vi "Main Module.vi"(8 "Error In":errorcluster) -> (0 "Error Out":errorcluster)   [LabVIEW 2015, in "Entry Console.lvlib"]
uses:
  Entry Console.lvlib
  Public Controls/Wash steps selection buttons.ctl
  Private Controls/Module Data Cluster.ctl
  Private Controls/Module Action.ctl
  Controller/Controller.lvlib
panel:
  in  "Start":bool
  in  "Wash steps selection buttons":T1={"Under Body Wash"=FALSE, "Bug Remover"=FALSE, "Pre-Soak"=FALSE, "High Pressure Wash"=TRUE, "Low Pressure Wax"=FALSE, "Spot Free Rinse"=FALSE, "Tire Shine Foam"=FALSE, "Air Dry"=FALSE}
  # "[Covers: UI1]"
  # "[Covers: UI2]"
  # "[Covers: UI2A]"
  # "[Covers: UI2A1]"
  # "[Covers: UI2B]"
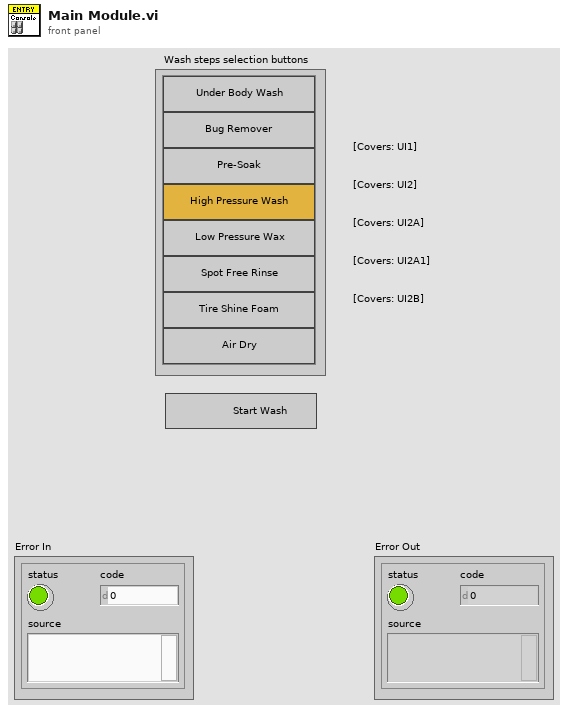
[diagram p1: front panel]
types:
  T1 = typedef "Entry Console.lvlib/Wash steps selection buttons.ctl" = cluster{"Under Body Wash":bool, "Bug Remover":bool, "Pre-Soak":bool, "High Pressure Wash":bool, "Low Pressure Wax":bool, "Spot Free Rinse":bool, "Tire Shine Foam":bool, "Air Dry":bool}
  T2 = typedef "Entry Console.lvlib/Module Data Cluster.ctl" = cluster{"Data":variant, "Action":T3}
  T3 = typedef "Entry Console.lvlib/Module Action.ctl" = enum16{"Init", "Close", "Error", "Start Wash"}
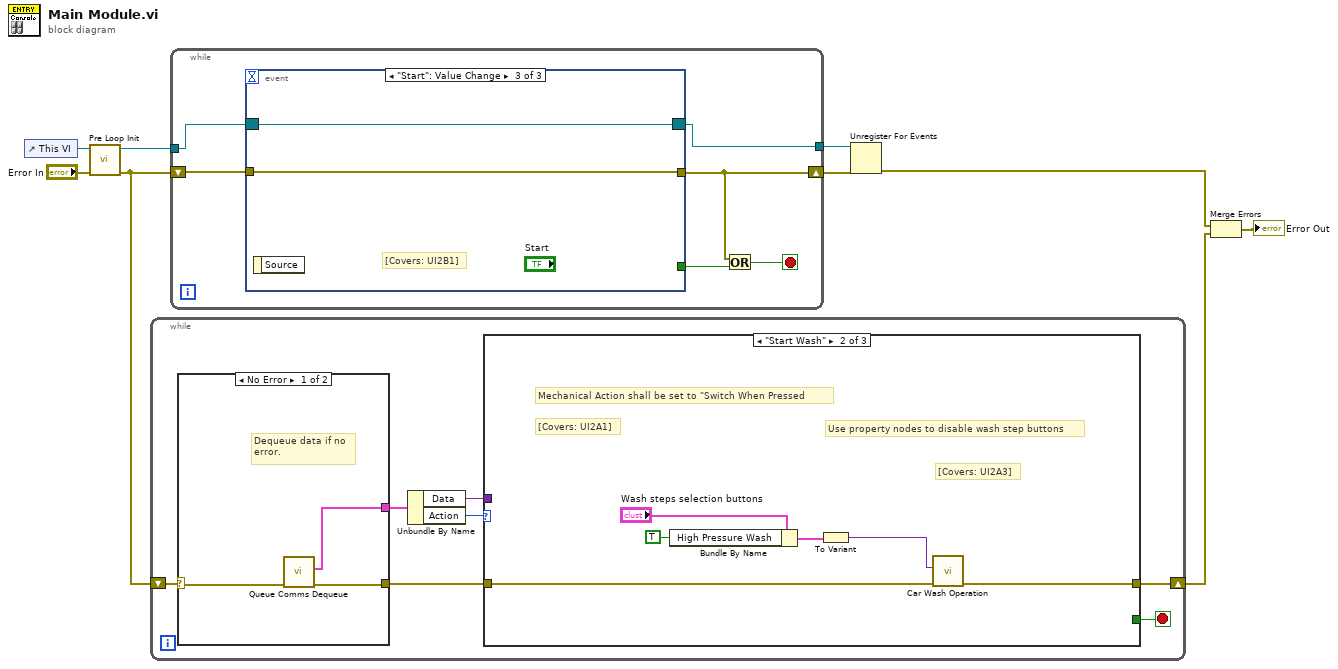
[diagram p0: block diagram]
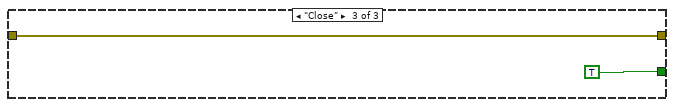
[diagram p3: hidden frame]
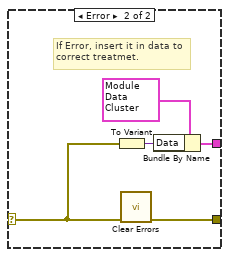
[diagram p4: hidden frame]
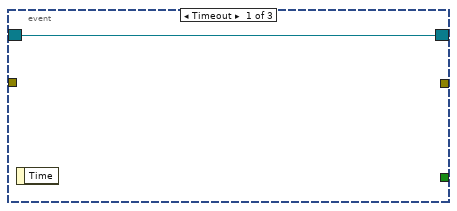
[diagram p5: hidden frame]
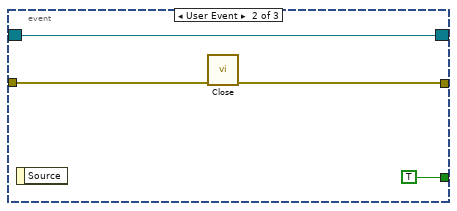
[diagram p6: hidden frame]
diagram:
  n1 = control-ref of="This VI"() -> (w8:refnum<vi>)
  n2 = call "Pre Loop Init.vi"("Error In"="Error In", "This VI"=w8) -> ("Error Out"=w4:errorcluster, "Event Registration Refnum"=w7:refnum<event-registration>)  [unwired: 8 in]
  n3 = while {
    shift-right: [w10] -> w2
    shift-left: w4 -> [w16]
    stop <- w11 stop-if-true
    n4 = case shown="No Error" w16 {
      selector: w16 -> [w28 w31]
      tunnel: [w27 w30] -> w13
      tunnel: [w26 w29] -> w15
      frame No Error {
        # "Dequeue data if no\nerror."
        n5 = call "Queue Comms Dequeue.vi"("Error In"=w28) -> ("Error Out"=w27:errorcluster, "Message Data"=w26:T2)  [unwired: 9 in]
      }
      frame Error {
        # "If Error, insert it in data to\ncorrect treatmet."
        n6 = To Variant(anything=w31) -> (Variant=w32:variant)
        n7 = call <vilib>:"Clear Errors.vi"("error in (no error)"=w31) -> ("error out"=w30:errorcluster)  [unwired: 5 in, 1 out]
        n8 = Bundle By Name(cluster=T2 {"Data"=variant, "Action"=enum."Error"} ("Message Data"), "Data"=w32) -> (w29:T2)
      }
    }
    n9 = Unbundle By Name(w15) -> ("Data"=w12:variant, "Action"=w14:T3)
    n10 = case shown="\"Start Wash\"" w14 {
      tunnel: w13 -> [w17 w21 w24]
      tunnel: w12 -> [_ _ _]
      tunnel: [_ _ TRUE] -> w11
      tunnel: [w17 w20 w24] -> w10
      frame "Init", Default {
      }
      frame "Start Wash" {
        # "Use property nodes to disable wash step buttons"
        # "[Covers: UI2A3]"
        # "Mechanical Action shall be set to \"Switch When Pressed"
        # "[Covers: UI2A1]"
        n11 = Bundle By Name(cluster="Wash steps selection buttons", "High Pressure Wash"=TRUE) -> (w19:T1)
        n12 = To Variant(anything=w19) -> (Variant=w18:variant)
        n13 = call "Car Wash Operation.vi"("Error In"=w21, "Data"=w18) -> ("Error Out"=w20:errorcluster)  [unwired: 9 in]
      }
      frame "Close" {
      }
    }
  }
  n14 = while {
    tunnel: w7 -> [w39]
    shift-right: [w36] -> w6
    shift-left: w4 -> [w37]
    tunnel: [w34] -> w5
    stop <- w38 stop-if-true
    n15 = event shown="[2] \"Start\": Value Change" {
      selector: w39 -> [w40 w44 w46]
      dyn-events: [w40 w44 w46] -> w34
      timeout: _ -> [_ _ _]
      tunnel: [_ w42 w45] -> w36
      tunnel: w37 -> [_ w43 w45]
      tunnel: [_ TRUE _] -> w35
      event Timeout {
        n16 = event-data() -> ()  [unwired: 1 in, 1 out]
      }
      event User Event {
        n17 = event-data() -> ()  [unwired: 1 in, 1 out]
        n18 = call "Close.vi"("Error In"=w43) -> ("Error Out"=w42:errorcluster)  [unwired: 10 in]
      }
      event "Start": Value Change {
        # "[Covers: UI2B1]"
        n19 = event-data() -> ()  [unwired: 1 in, 1 out]
      }
    }
    n20 = Or(x=w36, y=w35) -> (x .or. y?=w38:bool)
  }
  n21 = Unregister For Events(event registration refnum=w5, error in=w6) -> (error out=w1:errorcluster)
  n22 = Merge Errors(w1, w2) -> (→"Error Out":errorcluster)
